vi "Set IConfiguration.vi"(10 "IConfiguration":refnum<class "IConfiguration.lvclass">, 11 "PCAN-USB Read-Write Raw CAN Frame Strategy in":refnum<class "PCAN-USB Base Strategy.lvclass">) -> (3 "PCAN-USB Read-Write Raw CAN Frame Strategy out":refnum<class "PCAN-USB Base Strategy.lvclass">)   [LabVIEW 2024, in "PCAN-USB Base Strategy.lvclass"]
uses:
  PCAN-USB Base Strategy.lvclass
  Source/Interfaces/IConfiguration/IConfiguration.lvclass
  PCAN-USB Base Strategy.lvclass/PCAN-USB Base Strategy.ctl
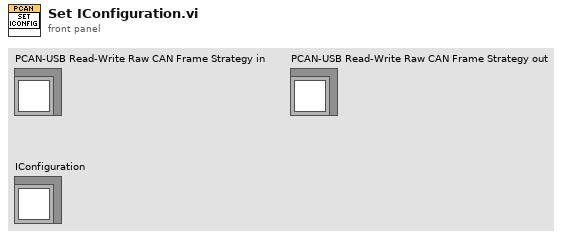
[diagram p1: front panel]
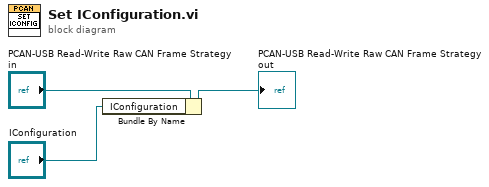
[diagram p0: block diagram]
diagram:
  n1 = Bundle By Name(cluster="PCAN-USB Read-Write Raw CAN Frame Strategy in", "IConfiguration"="IConfiguration") -> (→"PCAN-USB Read-Write Raw CAN Frame Strategy out":refnum<class "PCAN-USB Base Strategy.lvclass">)
